vi "LABVIEW_ATMEGA_robot_control.vi"() -> ()   [LabVIEW 2013]
doc: "This example performs writes and reads on a serial port, as directed by the user. You can press the Write and Read buttons, and change the Read Count, while the example is running.\n\nThe parameters set for the serial port must match the parameters of the connected instrument or device. In this example, the Read Count parameter specifies the number of bytes that the serial port reads. If there were more bytes at the port than the specified number, those bytes would not be read. If there were less bytes at the port than the specified number, you would receive a timeout error.\n\nThis example expands upon the flow control options for XON and XOFF, allowing the user to choose those control characters. Also, the user can enable or disable a termination character. Some devices require a termination character in order to identify the end of command strings. Some devices send a termination character to signify the end of data to be read. This example shows how you can end the Read operation once a termination character is detected in the buffer and/or append a termination character at the end of the Write data."
uses:
  D:/Program Files (x86)/National Instruments/LabVIEW 2013/examples/Instrument IO/Serial/support/Serial - Settings.ctl
  <vilib>/Instr/_visa.llb/VISA Configure Serial Port (Instr).vi
panel:
  in  "STOP":bool
  in  "RIGHT":bool
  in  "LEFT":bool
  in  "REVERSE":bool
  in  "Stop":bool
  in  "FORWARD":bool
  in  "Serial Settings":T1={"baud rate"=9600, "data bits"=8, "parity"=enum."None", "stop bits"=10, "flow control"=0} {"flow control" items=["None"=0, "XON/XOFF"=1, "RTS/CTS"=2, "DTR/DSR"=4]; "stop bits" items=["1.0"=10, "1.5"=15, "2.0"=20]; "data bits" min=5 max=8 step=1; "baud rate" items=["75"=75, "110"=110, "134"=134, "150"=150, "300"=300, "600"=600, "1200"=1200, "1800"=1800, "2400"=2400, "4800"=4800, "7200"=7200, "9600"=9600, "14400"=14400, "19200"=19200, "28800"=28800, "38400"=38400, "56000"=56000, "57600"=57600, "115200"=115200, "128000"=128000, "230400"=230400]}
  in  "VISA resource name":refnum<visa-resource-name>="COM1"
  # "Overview: Demonstrates the use of the VISA functions to write commands to and read responses from a serial instrument continuously in a loop.\nRequirements: NI-VISA Driver\nInstructions:\n1. Run the VI.\n2. Specify a Command and click the Write button.\n3. Read a Response by clicking the Read button.\n4. Click Stop to stop the VI."
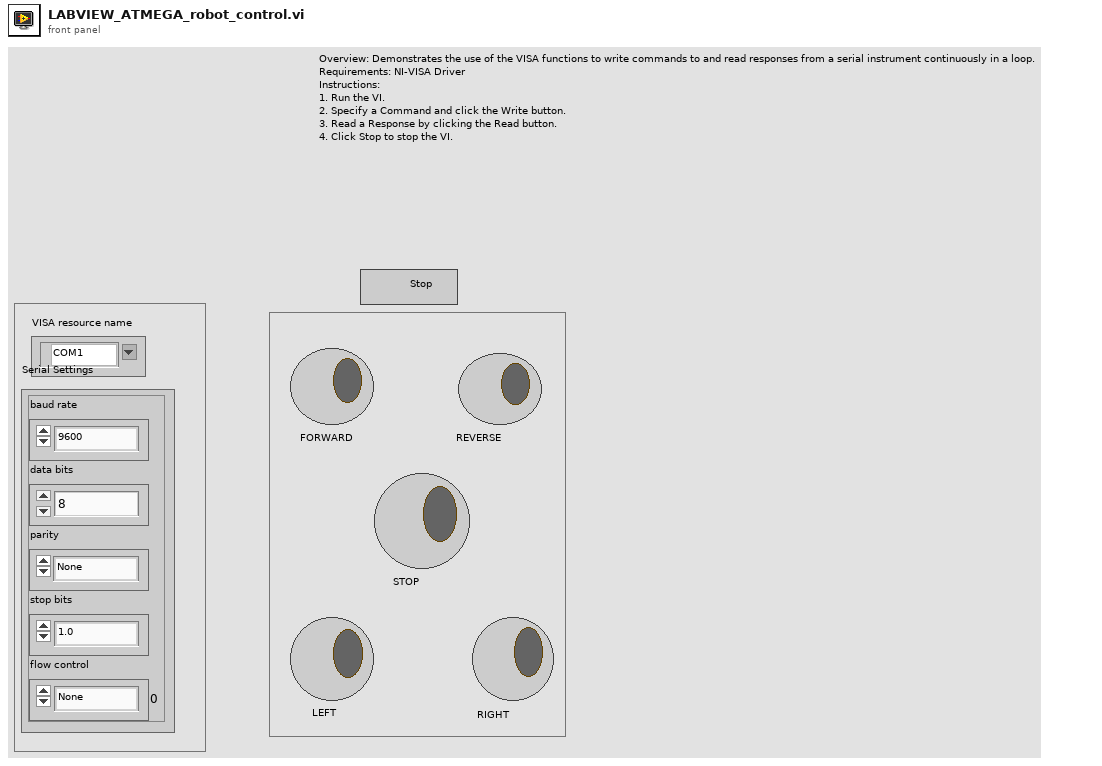
[diagram p1: front panel]
types:
  T1 = typedef "Serial - Settings.ctl" = cluster{"baud rate":u32, "data bits":u16, "parity":enum16{"None", "Odd", "Even", "Mark", "Space"}, "stop bits":u16, "flow control":u16}
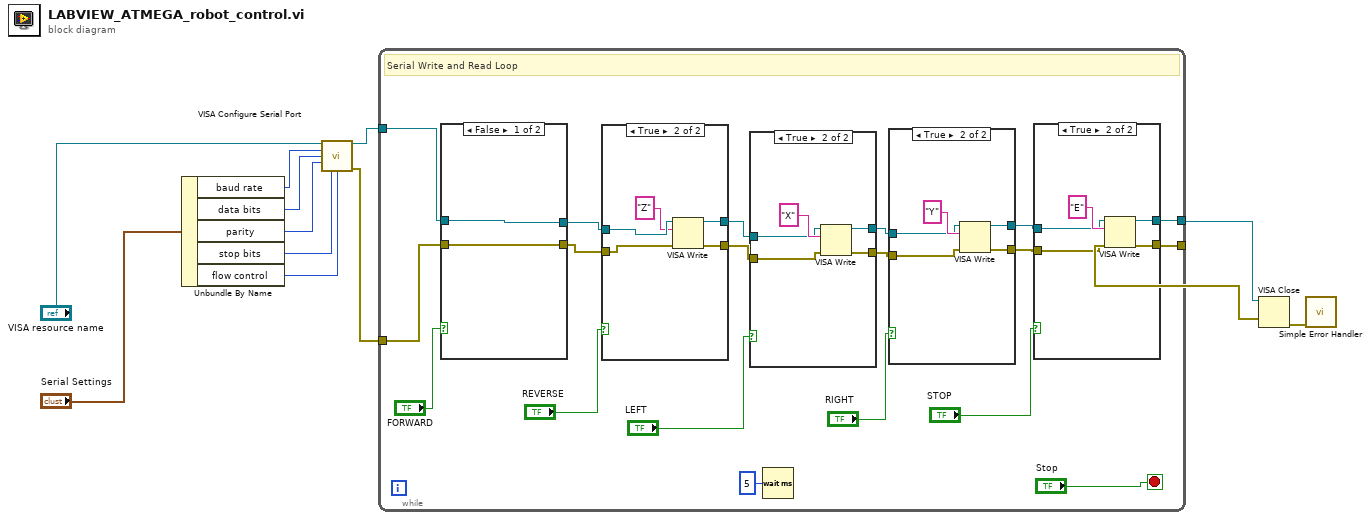
[diagram p0: block diagram]
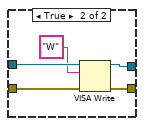
[diagram p6: hidden frame]
diagram:
  n1 = Unbundle By Name "Unbundle By Name"("Serial Settings") -> ("baud rate"=w8:u32, "data bits"=w9:u16, "parity"=w10:enum16{"None", "Odd", "Even", "Mark", "Space"}, "stop bits"=w11:u16, "flow control"=w5:u16)
  n2 = call-poly "VISA Configure Serial Port"("VISA resource name"="VISA resource name", "baud rate (9600)"=w8, "data bits (8)"=w9, "parity (0:none)"=w10, "stop bits (10: 1 bit)"=w11, "flow control (0:none)"=w5) -> ("VISA resource name out"=w3:refnum<visa-resource-name>, "error out"=w4:errorcluster)  [unwired: 4 in, 4 out]
  n3 = while {
    tunnel: w4 -> [w30]
    tunnel: w3 -> [w27]
    tunnel: [w18] -> w2
    tunnel: [w19] -> w1
    stop <- "Stop" stop-if-true
    # "Serial Write and Read Loop"
    n4 = case shown="False" "FORWARD" {
      tunnel: w27 -> [w61 w66]
      tunnel: w30 -> [w60 w65]
      tunnel: [w61 w64] -> w28
      tunnel: [w60 w63] -> w29
      frame False {
      }
      frame True {
        n5 = VISA Write(VISA resource name=w66, write buffer="W", error in (no error)=w65) -> (VISA resource name out=w64:refnum<visa-resource-name>, error out=w63:errorcluster)  [unwired: 1 out]
      }
    }
    n6 = case shown="True" "REVERSE" {
      tunnel: [w54 w59] -> w25
      tunnel: [w53 w58] -> w24
      tunnel: w29 -> [w53 w57]
      tunnel: w28 -> [w54 w56]
      frame False {
      }
      frame True {
        n7 = VISA Write(VISA resource name=w56, write buffer="Z", error in (no error)=w57) -> (VISA resource name out=w59:refnum<visa-resource-name>, error out=w58:errorcluster)  [unwired: 1 out]
      }
    }
    n8 = case shown="True" "LEFT" {
      tunnel: [w47 w52] -> w23
      tunnel: [w46 w51] -> w22
      tunnel: w24 -> [w46 w48]
      tunnel: w25 -> [w47 w49]
      frame False {
      }
      frame True {
        n9 = VISA Write(VISA resource name=w49, write buffer="X", error in (no error)=w48) -> (VISA resource name out=w52:refnum<visa-resource-name>, error out=w51:errorcluster)  [unwired: 1 out]
      }
    }
    n10 = Wait (ms)(milliseconds to wait=u32 5) -> ()  [unwired: 1 out]
    n11 = case shown="True" "RIGHT" {
      tunnel: [w40 w45] -> w21
      tunnel: [w39 w44] -> w20
      tunnel: w22 -> [w39 w41]
      tunnel: w23 -> [w40 w42]
      frame False {
      }
      frame True {
        n12 = VISA Write(VISA resource name=w42, write buffer="Y", error in (no error)=w41) -> (VISA resource name out=w45:refnum<visa-resource-name>, error out=w44:errorcluster)  [unwired: 1 out]
      }
    }
    n13 = case shown="True" "STOP" {
      tunnel: [w33 w38] -> w19
      tunnel: [w32 w37] -> w18
      tunnel: w20 -> [w32 w34]
      tunnel: w21 -> [w33 w35]
      frame False {
      }
      frame True {
        n14 = VISA Write(VISA resource name=w35, write buffer="E", error in (no error)=w34) -> (VISA resource name out=w38:refnum<visa-resource-name>, error out=w37:errorcluster)  [unwired: 1 out]
      }
    }
  }
  n15 = VISA Close(VISA resource name=w1, error in (no error)=w2) -> (error out=w6:errorcluster)
  n16 = call <vilib>:"Simple Error Handler.vi"("error in (no error)"=w6) -> ()  [unwired: 1 in, 8 out]
